vi "MedianFilter_Example.vi"() -> ()   [LabVIEW 2019]
uses:
  <vilib>/Rock Robotics/WPI/ThirdParty/JAS_Junk/TrajLib/MedianFilter_New.vi
  <vilib>/Rock Robotics/WPI/ThirdParty/JAS_Junk/TrajLib/MedianFilter_ResetToValue.vi
  <vilib>/Rock Robotics/WPI/ThirdParty/JAS_Junk/TrajLib/MathUtil_Clamp.vi
  <vilib>/Rock Robotics/WPI/ThirdParty/JAS_Junk/TrajLib/MedianFilter_Calculate.vi
  <vilib>/Rock Robotics/WPI/ThirdParty/JAS_Junk/TrajLib/Trajectory_Library.lvlib
panel:
  out "Wait Adjust":dbl format="%11.3f"
  in  "Auto / Manual":bool=TRUE
  in  "Enable\nNoise":bool=TRUE
  in  "Filter Enable":bool=TRUE
  in  "Use White Noise":bool=TRUE
  in  "Tab Control 2":enum32{"Med 3", "Med 7"}(tab)
  out "Med3":cluster{dbl, dbl, "Value_Output":dbl}(graph)
  out "Med3 Out":dbl format="%11.3f"
  out "Med3 Out Dial":dbl(knob)=-2.895988890827539e-05 scale=-20.0..20.0
  out "Med7":cluster{dbl, dbl, "Value_Output":dbl}(graph)
  out "Med7 Out":dbl format="%11.3f"
  out "Med7 Out Dial":dbl(knob)=-2.895988890827539e-05 scale=-20.0..20.0
  out "Duration":dbl format="%11.3f"
  out "Late":dbl format="%11.3f"
  in  "Manual\nInput":dbl(slide) min=-12.0 max=12.0 scale=-12.0..12.0
  out "Raw Noise":dbl(knob)=-2.895988890827539e-05 scale=-20.0..20.0
  out "Raw Noise":dbl format="%11.3f"
  out "Actual Input":dbl(knob)=-2.895988890827539e-05 scale=-20.0..20.0
  out "Actual Input":dbl format="%11.3f"
  out "Input":cluster{"Manual\nInput":dbl, dbl, "f":dbl}(graph)
  out "Meas Dial":dbl(knob)=-2.895988890827539e-05 scale=-20.0..20.0
  out "Measured Value":dbl format="%11.3f"
  # "Median Filter Example"
  # "Loop Execution"
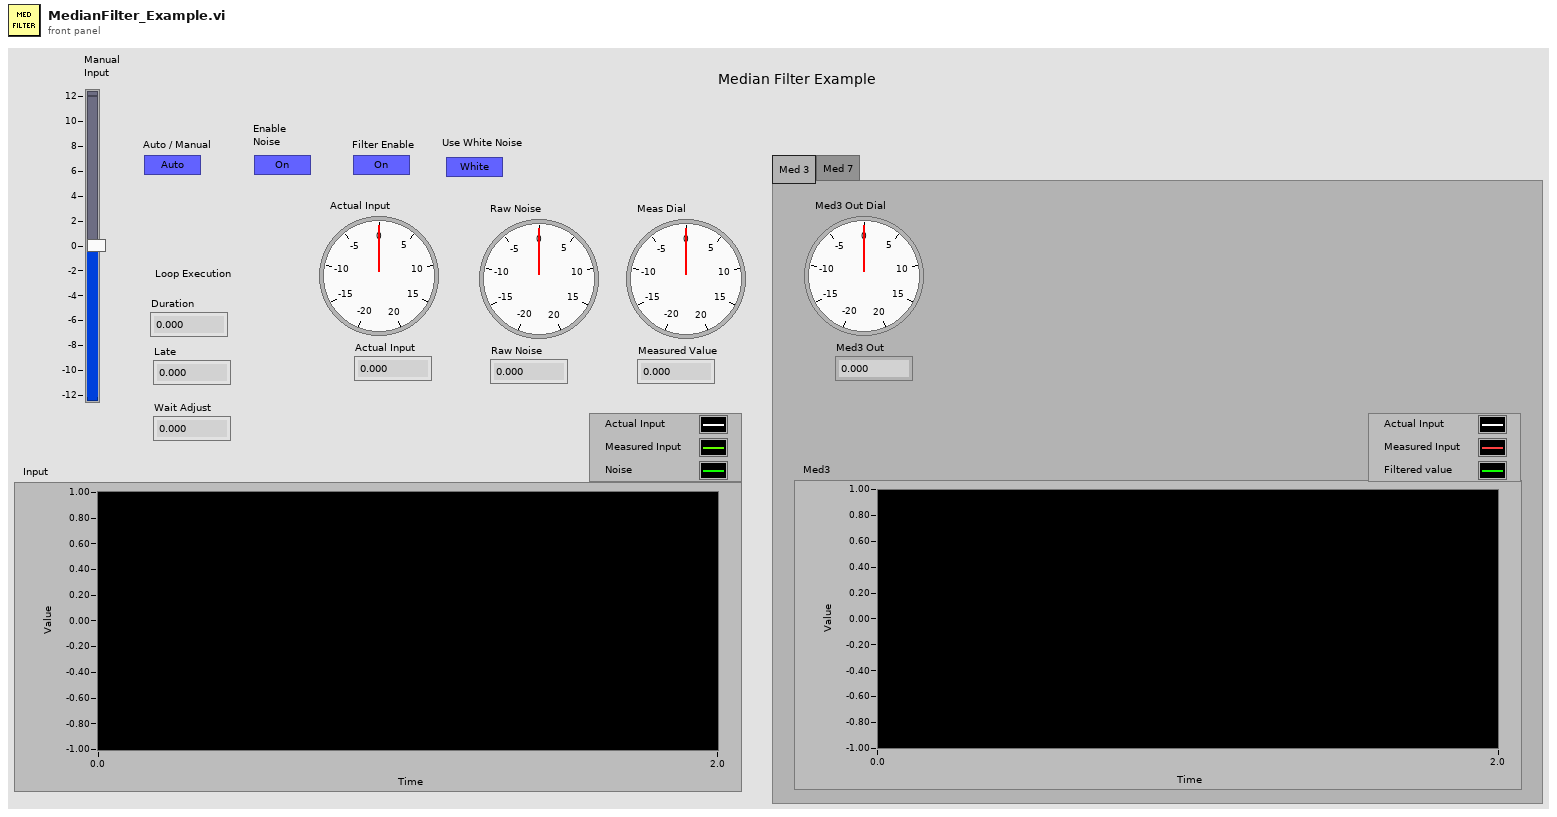
[diagram p1: front panel]
types:
  T1 = cluster{"Manual\nInput":dbl, dbl, "MedianValue":dbl}
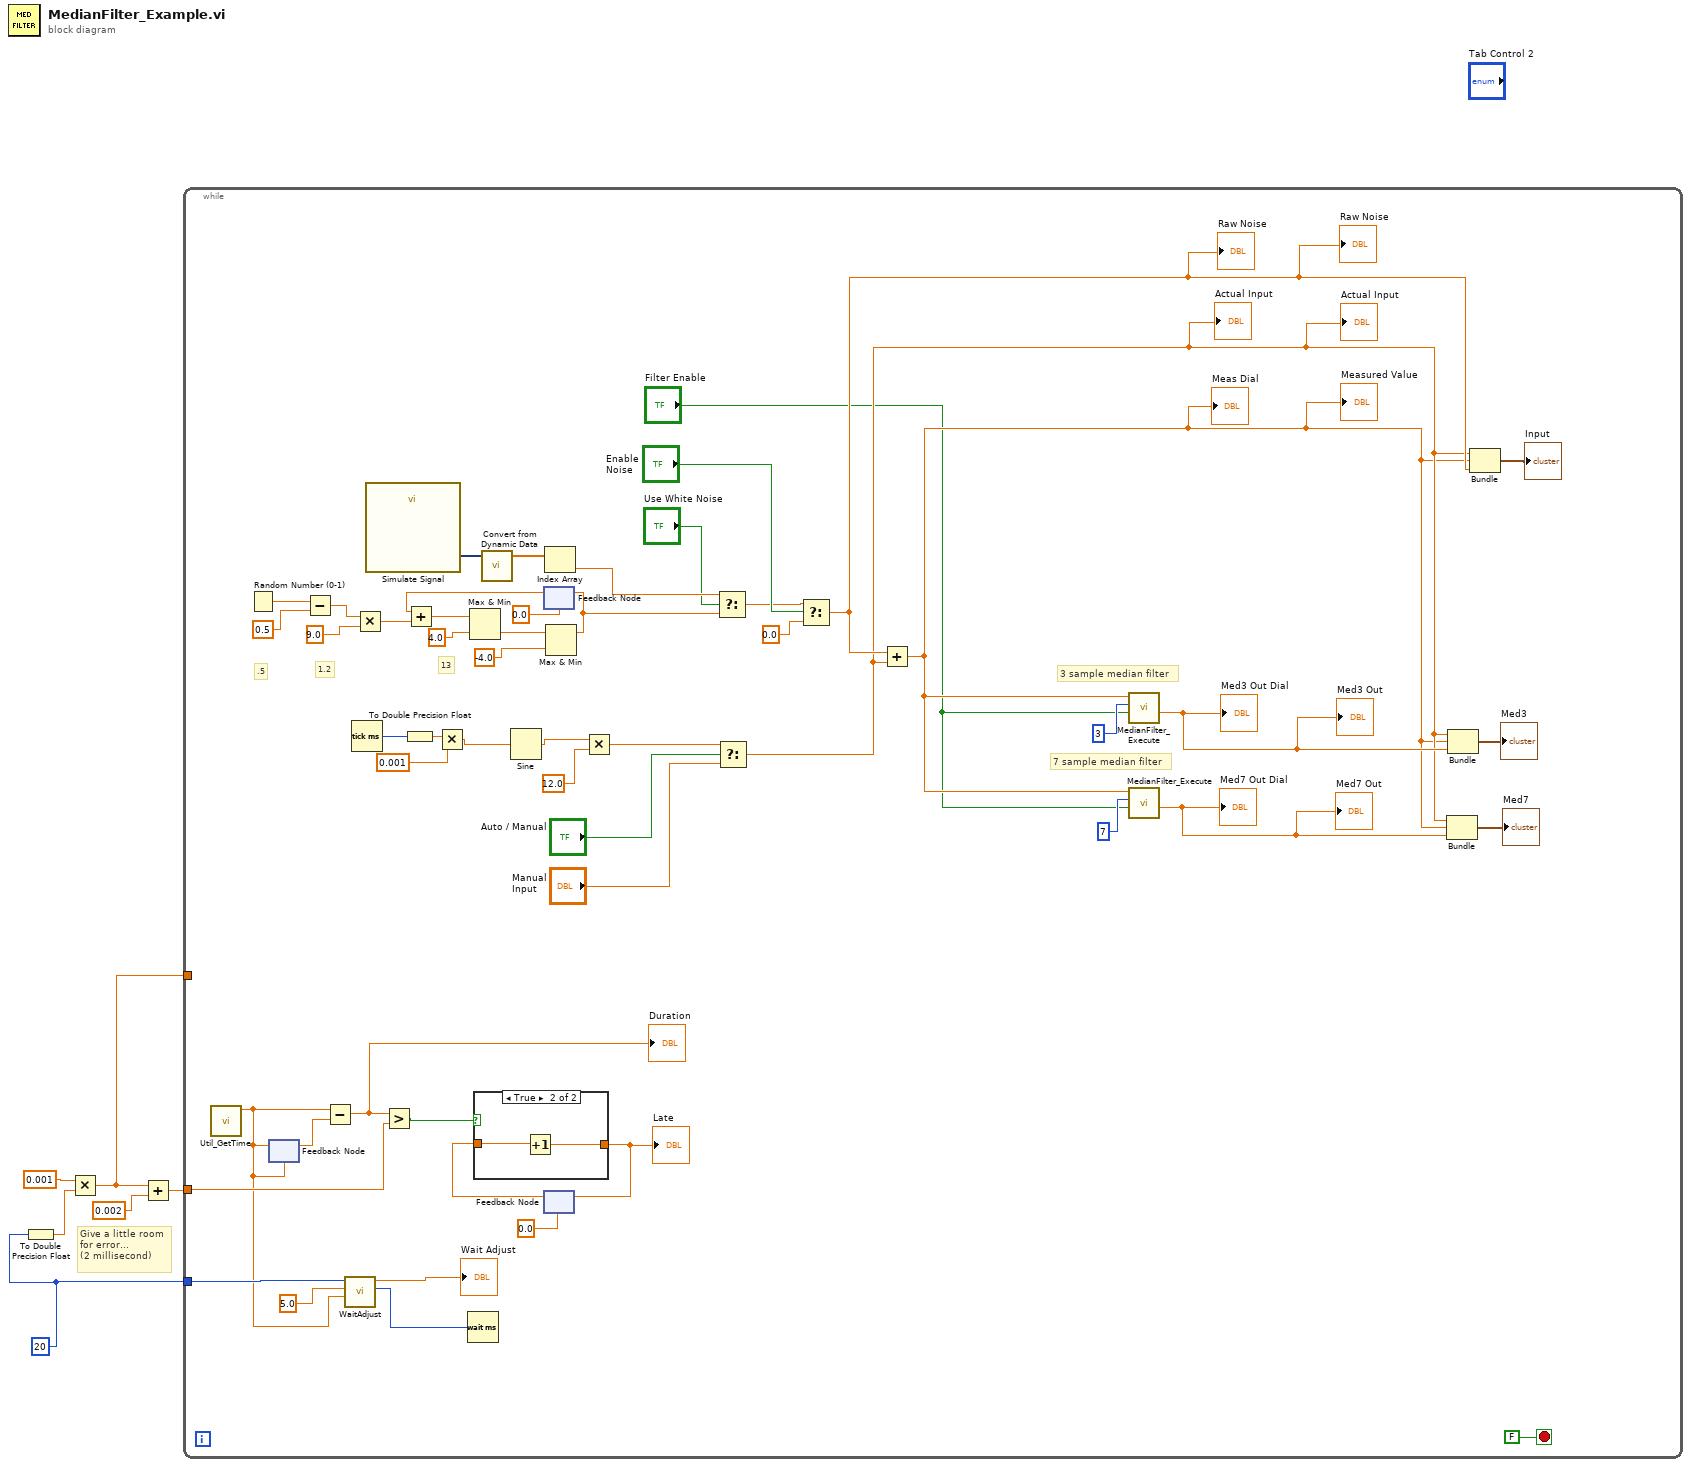
[diagram p0: block diagram]
diagram:
  w4 = u32 20 ("milliseconds to wait")
  # "Give a little room\nfor error...\n(2 millisecond)"
  n1 = To Double Precision Float(number=w4) -> (double precision float=w6:dbl)
  n2 = Multiply(x=0.001, y=w6) -> (x*y=w1:dbl)
  n3 = Add(x=w1, y=0.002) -> (x+y=w3:dbl)
  n4 = while {
    tunnel: w4 -> [w11]
    tunnel: w3 -> [w19]
    tunnel: w1 -> [_]
    stop <- FALSE stop-if-true
    # "7 sample median filter"
    # "3 sample median filter"
    # "13"
    # "1.2"
    # ".5"
    n5 = call <vilib>:"Util_GetTime.vi"() -> ("FPGA_Time_Seconds"=w9:dbl)  [unwired: 10 in, 1 out]
    n6 = Random Number (0-1)() -> (number: 0 to 1=w53:dbl)
    n7 = feedback-in #1(w9) -> ()
    n8 = feedback #1(w9) -> (w22:dbl)
    n9 = Subtract(x=w53, y=0.5) -> (x-y=w49:dbl)
    n10 = Subtract(x=w9, y=w22) -> (x-y=w20:dbl)
    "Duration" <- w20
    n11 = call <vilib>:"WaitAdjust.vi"("Time_SEC"=w9, "MaxDeviation_MS"=5.0, "DesiredLoopTime_MS"=w11) -> ("AdjustedWaitTime_MS"=w7:u32, "Offset_MS"=→"Wait Adjust":dbl)  [unwired: 7 in]
    n12 = Tick Count (ms)() -> (millisecond timer value=w44:u32)
    n13 = Multiply(x=w49, y=9.0) -> (x*y=w48:dbl)
    n14 = call "Simulate Signal"() -> ("DC with Uniform Noise"=w32:dynamicdata)  [unwired: 14 in, 1 out]
    n15 = Greater?(x=w20, y=w19) -> (0:w21:bool)
    n16 = To Double Precision Float(number=w44) -> (double precision float=w45:dbl)
    n17 = Multiply(x=w45, y=0.001) -> (x*y=w42:dbl)
    n18 = Wait (ms)(milliseconds to wait=w7) -> ()  [unwired: 1 out]
    n19 = call "Convert from Dynamic Data"("Dynamic Data Type"=w32) -> ("Array"=w31:dbl[])  [unwired: 3 in]
    n20 = Sine(x=w42) -> (sin(x)=w41:dbl)
    n21 = feedback #2(0.0) -> (w50:dbl)
    n22 = Add(x=w50, y=w48) -> (x+y=w52:dbl)
    n23 = Max & Min(x=w52, y=4.0) -> (min(x,y)=w51:dbl)  [unwired: 1 out]
    n24 = feedback #3(0.0) -> (w25:dbl)
    n25 = case shown="True" w21 {
      tunnel: [w59 w61] -> w26
      tunnel: w25 -> [w59 w60]
      frame False {
      }
      frame True {
        n26 = Increment(x=w60) -> (x+1=w61:dbl)
      }
    }
    "Late" <- w26
    n27 = feedback-in #3(w26) -> ()
    n28 = Index Array(array=w31) -> (element=w30:dbl)  [unwired: 1 in]
    n29 = Max & Min(x=w51, y=-4.0) -> (max(x,y)=w33:dbl)  [unwired: 1 out]
    n30 = feedback-in #2(w33) -> ()
    n31 = Multiply(x=w41, y=12.0) -> (x*y=w38:dbl)
    n32 = Select(t=w30, s="Use White Noise", f=w33) -> (s? t:f=w34:dbl)
    n33 = Select(t=w38, s="Auto / Manual", f="Manual\nInput") -> (s? t:f=w14:dbl)
    "Actual Input" <- w14
    "Actual Input" <- w14
    n34 = Select(t=w34, s="Enable\nNoise", f=0.0) -> (s? t:f=w28:dbl)
    "Raw Noise" <- w28
    "Raw Noise" <- w28
    n35 = Add(x=w28, y=w14) -> (x+y=w13:dbl)
    "Measured Value" <- w13
    "Meas Dial" <- w13
    n36 = call <vilib>:"MedianFilter_Execute.vi"("Enable"="Filter Enable", "Samples"=3, "Input Value"=w13) -> ("MedianValue"=w16:dbl)  [unwired: 7 in, 1 out]
    "Med3 Out" <- w16
    "Med3 Out Dial" <- w16
    n37 = call <vilib>:"MedianFilter_Execute.vi"("Enable"="Filter Enable", "Samples"=7, "Input Value"=w13) -> ("MedianValue"=w18:dbl)  [unwired: 7 in, 1 out]
    "Med7 Out" <- w18
    "Med7 Out Dial" <- w18
    n38 = Bundle("Manual\nInput"=w14, w13, "MedianValue"=w18) -> (→"Med7":T1)  [unwired: 1 in]
    n39 = Bundle("Manual\nInput"=w14, w13, "MedianValue"=w16) -> (→"Med3":T1)  [unwired: 1 in]
    n40 = Bundle("Manual\nInput"=w14, w13, "f"=w28) -> (→"Input":cluster{"Manual\nInput":dbl, dbl, "f":dbl})  [unwired: 1 in]
  }
